vi "mainVI.vi"() -> ()   [LabVIEW 2017]
uses:
  Controls/ShiftRegisterCluster.ctl
  Controls/PhysicalChannelsArray.ctl
  Variables/GlobalData.vi
  <vilib>/regexp/Match Regular Expression.xnode
panel:
  in  "Remote start?":bool
  in  "VRMS simulation?":bool
  in  "VRMS Physical channel":tag caption="Physical channel"
  in  "DI simulation?":bool
  in  "Digital Input Lines":tag
  in  "Temp simulation?":bool
  in  "Temp physical channel":tag caption="Physical channel"
  out "IsAcqGoing":bool
  in  "StopAcqButton":bool
  in  "StartAcqButton":bool
  out "Frequency [Hz]":dbl format="%.2f"
  out "RMS Value [V]":dbl format="%0.2p"
  out "DI data":bool[](array[boolean])
  out "Temperature indicator":dbl caption="Temperature [°C]"
  in  "OK":bool
  # "Temperature"
  # "Digital Inputs"
  # "DAQ"
  # "Sim"
  # "DAQ"
  # "Sim"
  # "Voltage"
  # "DAQ"
  # "Sim"
  # "Remote"
  # "Loclal"
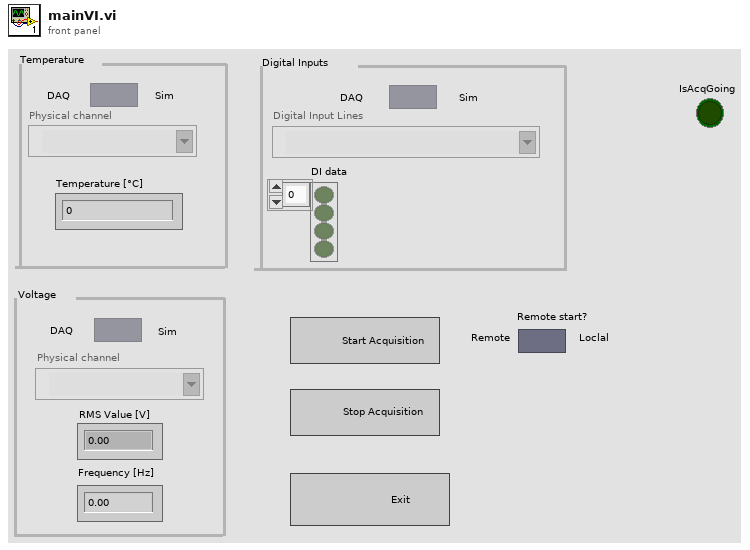
[diagram p1: front panel]
types:
  T1 = enum32{"invalid app kind", "Development System", "Run Time System", "Student Edition", "Embedded LabVIEW", "Evaluation", "Custom"}
  T2 = enum32{"Invalid", "Standard", "Closed", "Hidden", "Minimized", "Maximized"}
  T3 = enum8{"Enabled", "Disabled", "Disabled and Grayed Out"}
  T4 = typedef "ShiftRegisterCluster.ctl" = cluster{"TemperatureTask":refnum<k21>, "TemperatureData":dbl, "EncoderTask":refnum<k21>, "EncoderData":dbl, "DITask":refnum<k21>, "DIData":bool[], "VRMSTask":refnum<k21>, "VRMSData":dbl, "FreqData":dbl}
  T5 = cluster{"TemperatureData":dbl, "DIData":bool[], "VRMSData":dbl, "FreqData":dbl}
  T6 = cluster{"Core":cluster{"Current VI Reference":refnum<vi>, "Close Panel on Exit?":bool}, "Data Cluster":T4, "IsAcqGoing":bool}
  T7 = cluster{"Current VI Reference":refnum<vi>, "Close Panel on Exit?":bool}
  T8 = cluster{"Temp simulation?":bool, "DI simulation?":bool, "VRMS simulation?":bool}
  T9 = cluster{"Temp physical channel":tag, "Digital Input Lines":tag, "VRMS Physical channel":tag}
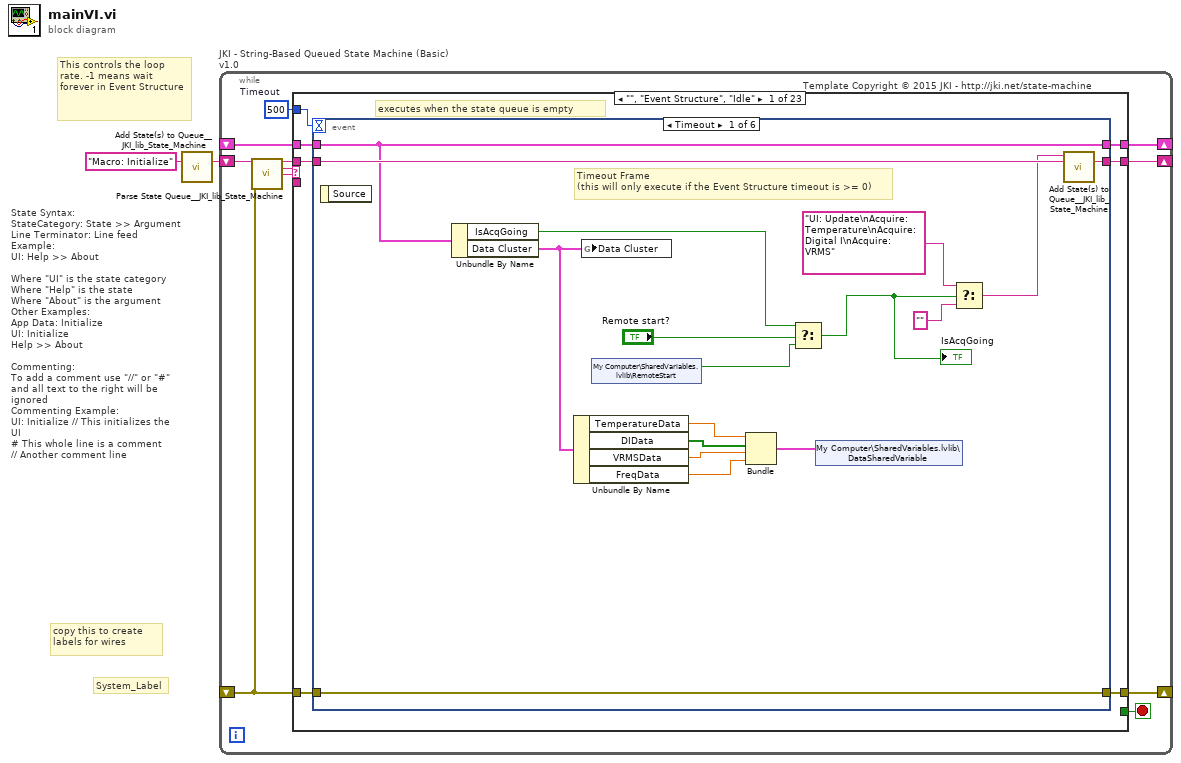
[diagram p0: block diagram]
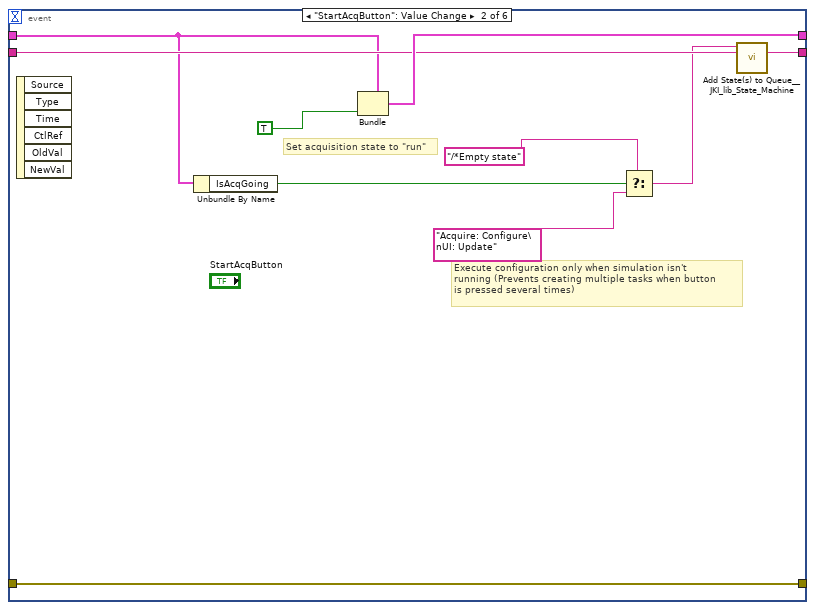
[diagram p2: hidden frame]
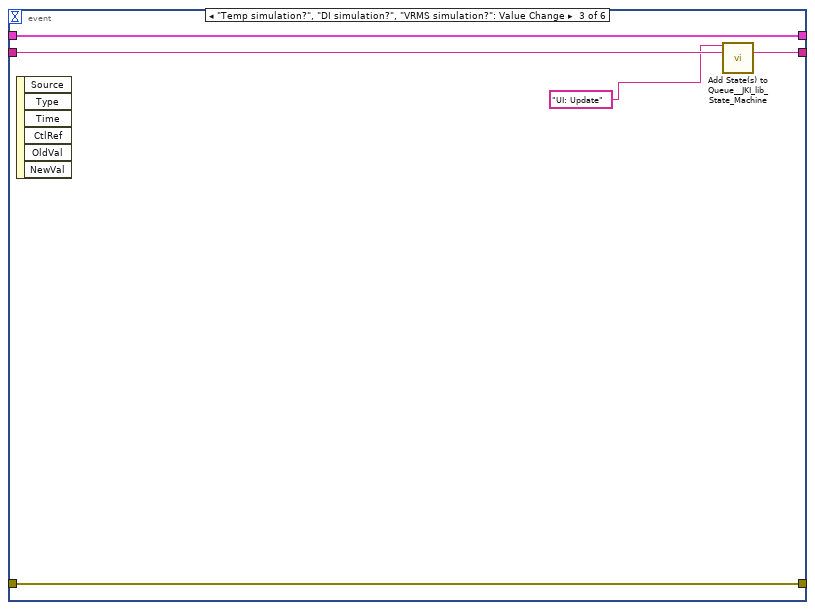
[diagram p3: hidden frame]
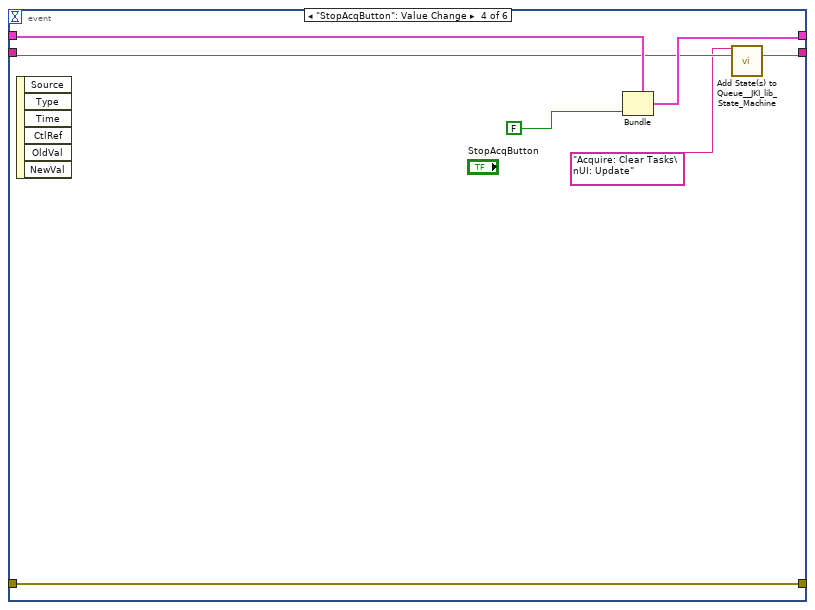
[diagram p4: hidden frame]
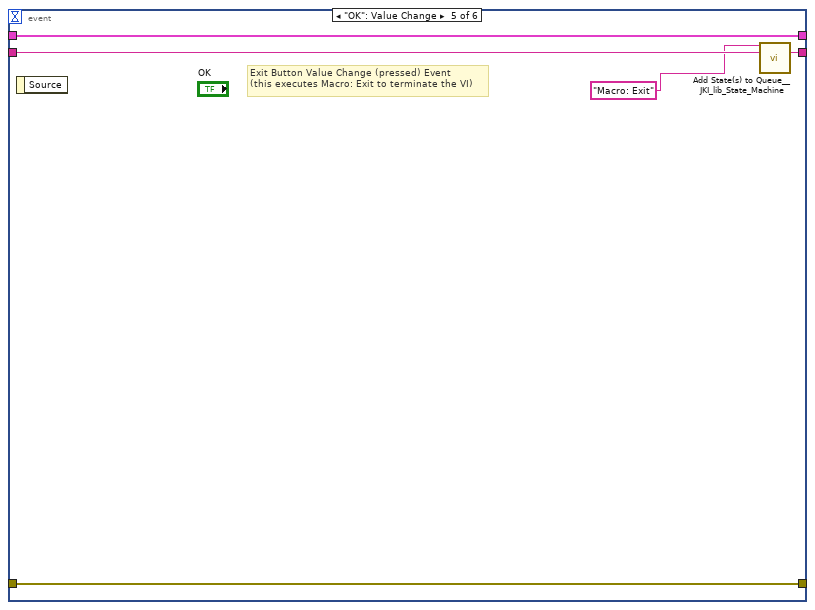
[diagram p5: hidden frame]
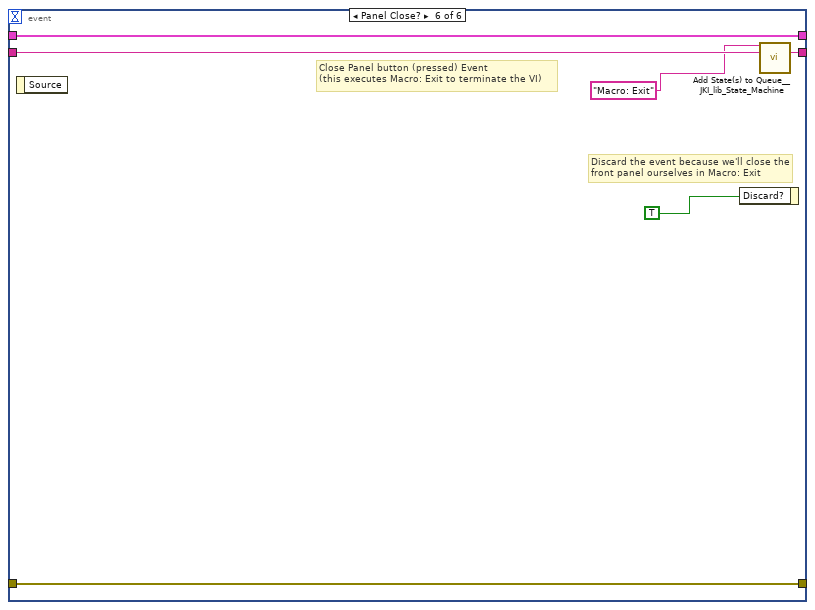
[diagram p6: hidden frame]
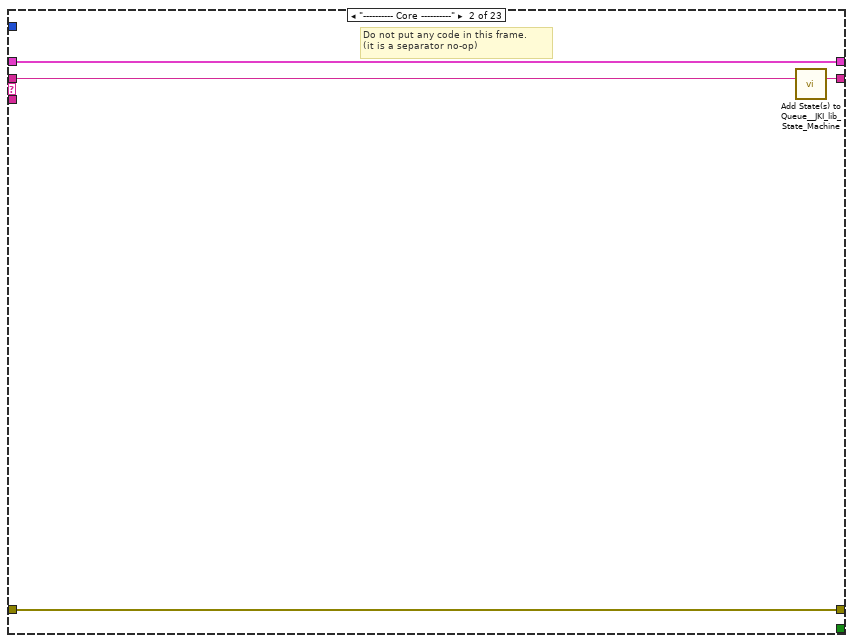
[diagram p7: hidden frame]
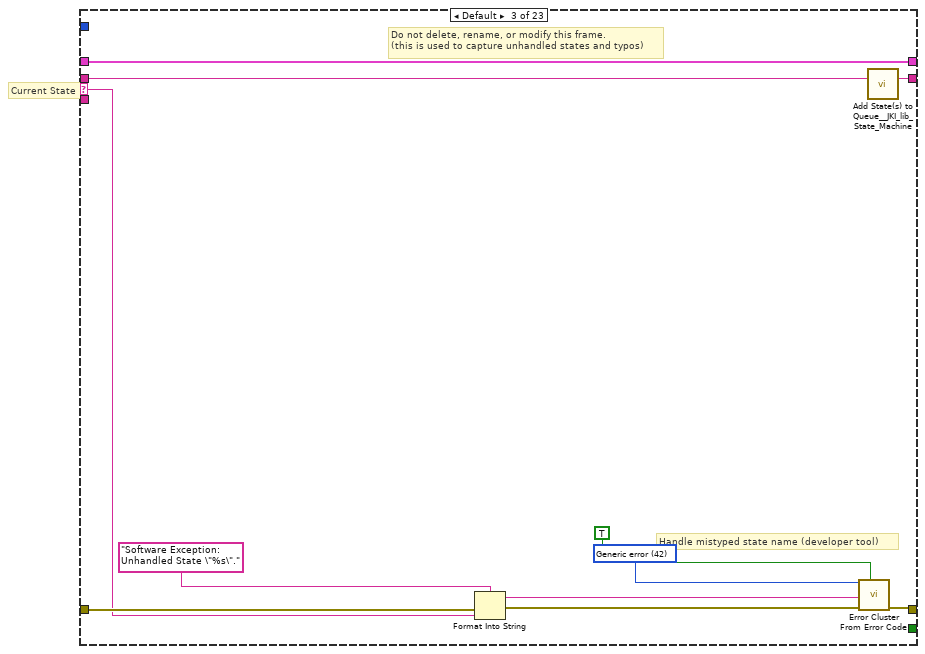
[diagram p8: hidden frame]
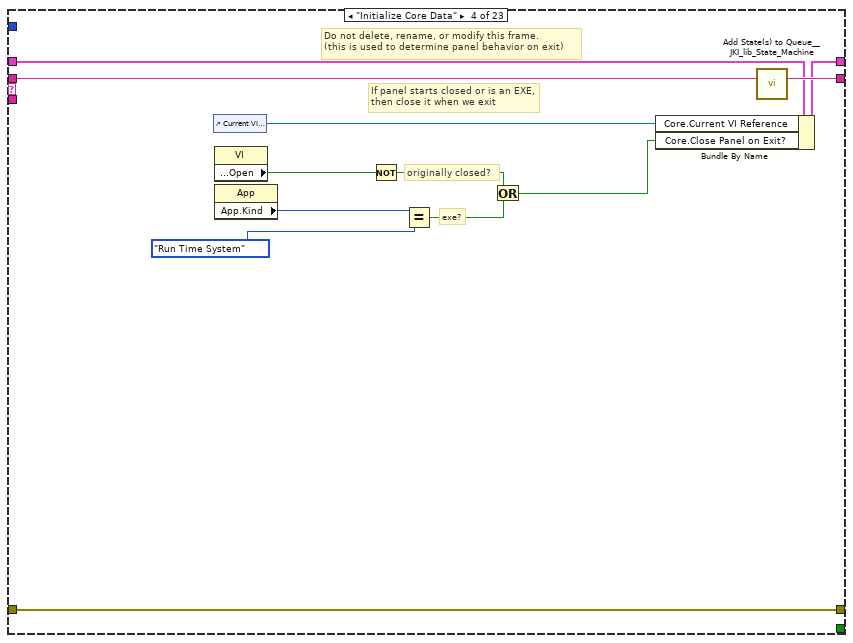
[diagram p9: hidden frame]
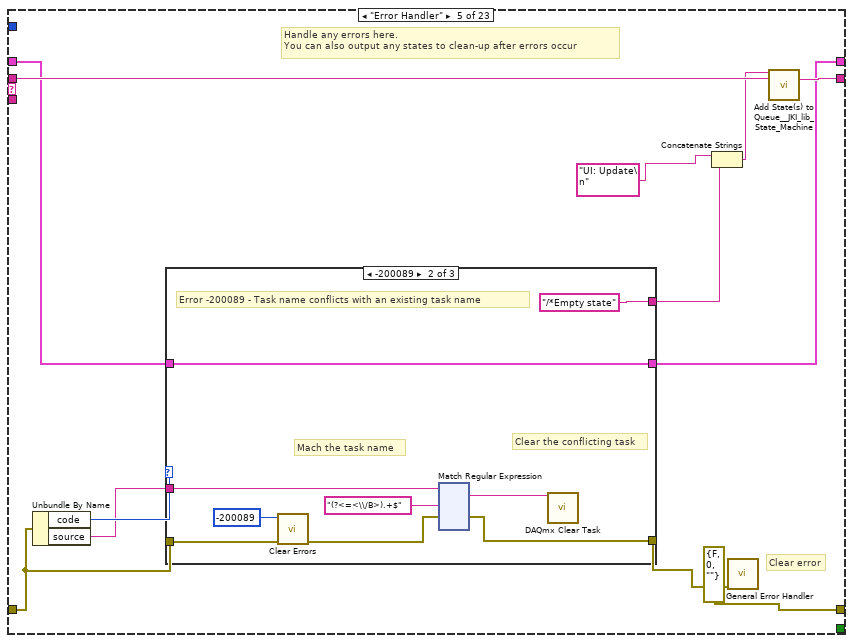
[diagram p10: hidden frame]
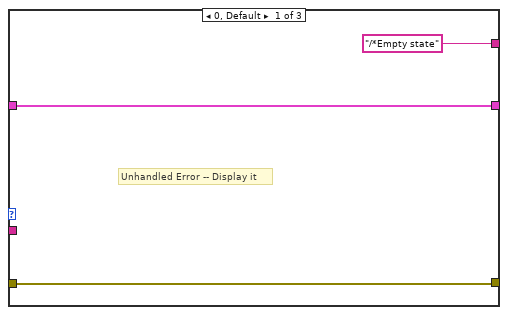
[diagram p11: hidden frame]
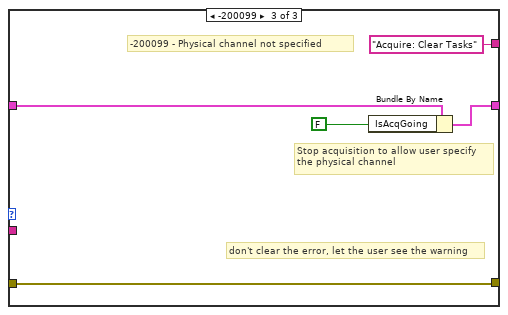
[diagram p12: hidden frame]
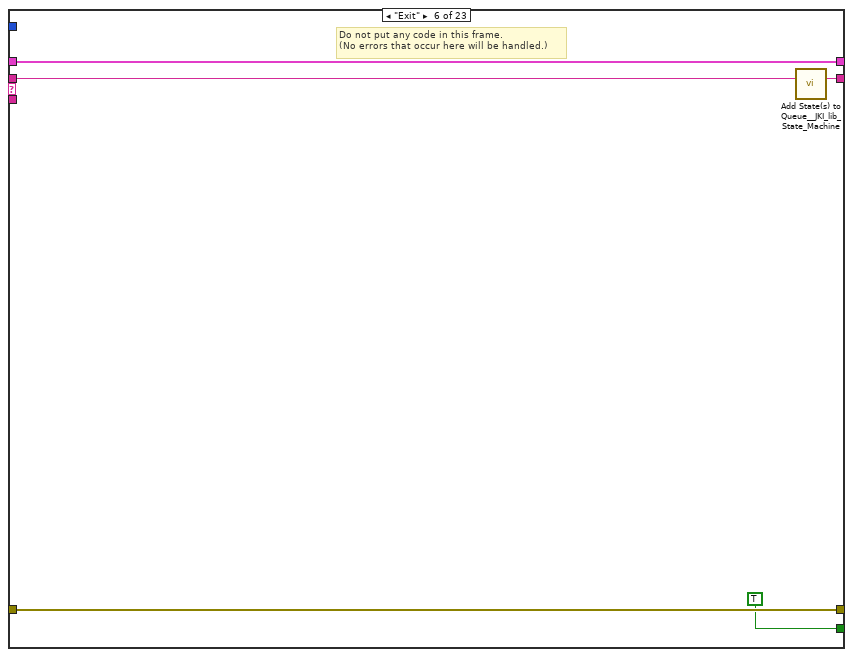
[diagram p13: hidden frame]
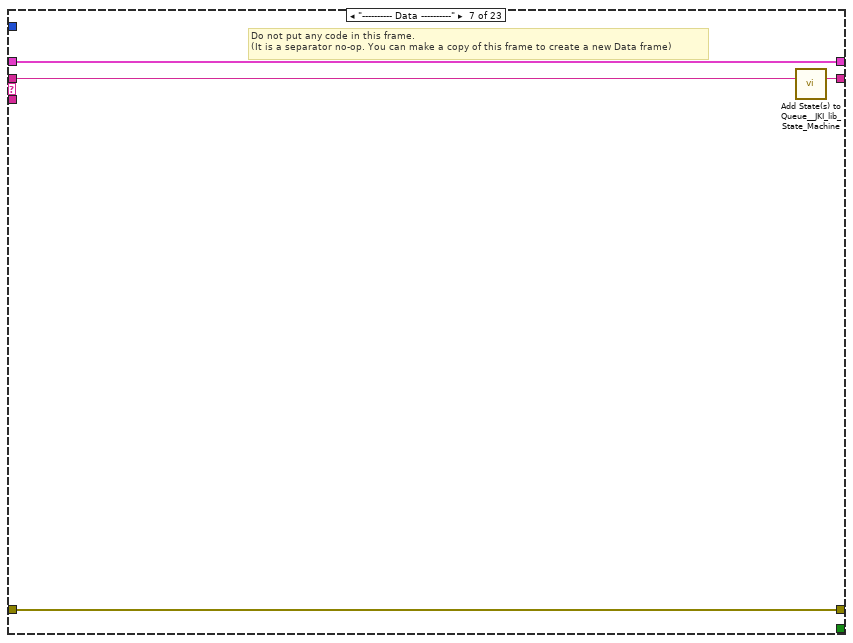
[diagram p14: hidden frame]
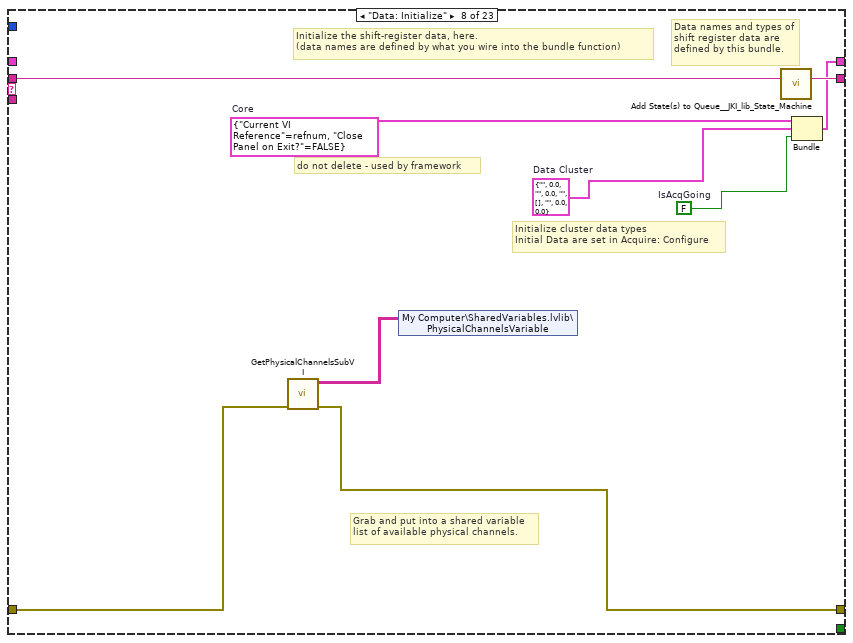
[diagram p15: hidden frame]
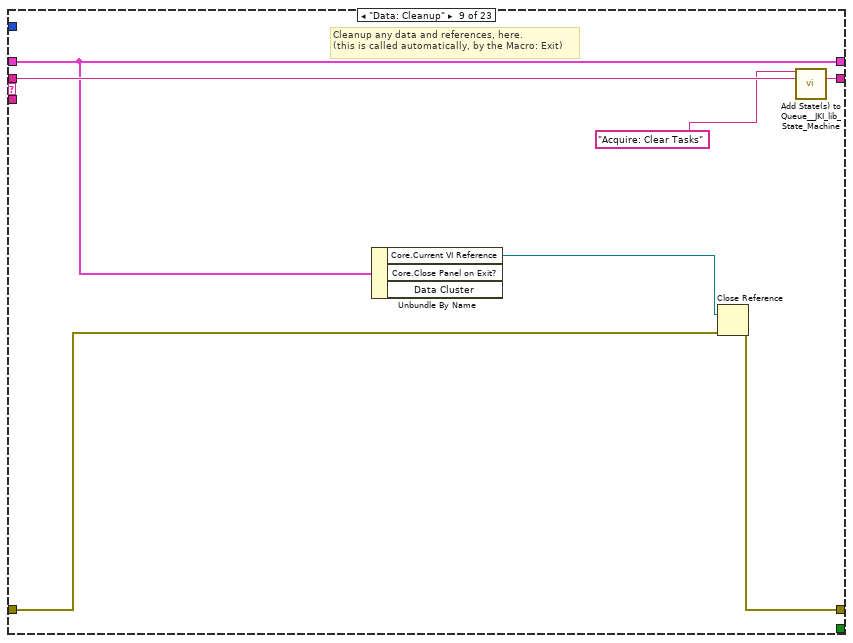
[diagram p16: hidden frame]
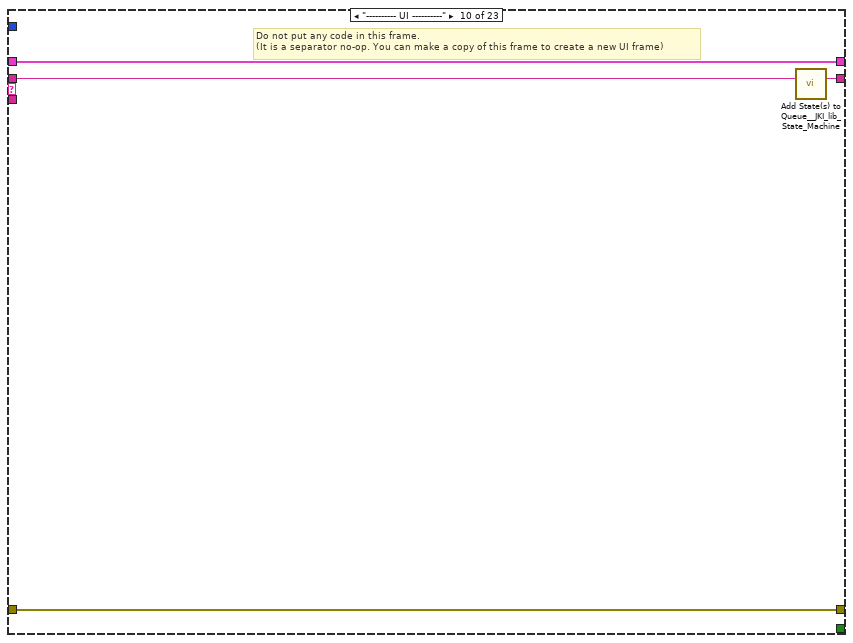
[diagram p17: hidden frame]
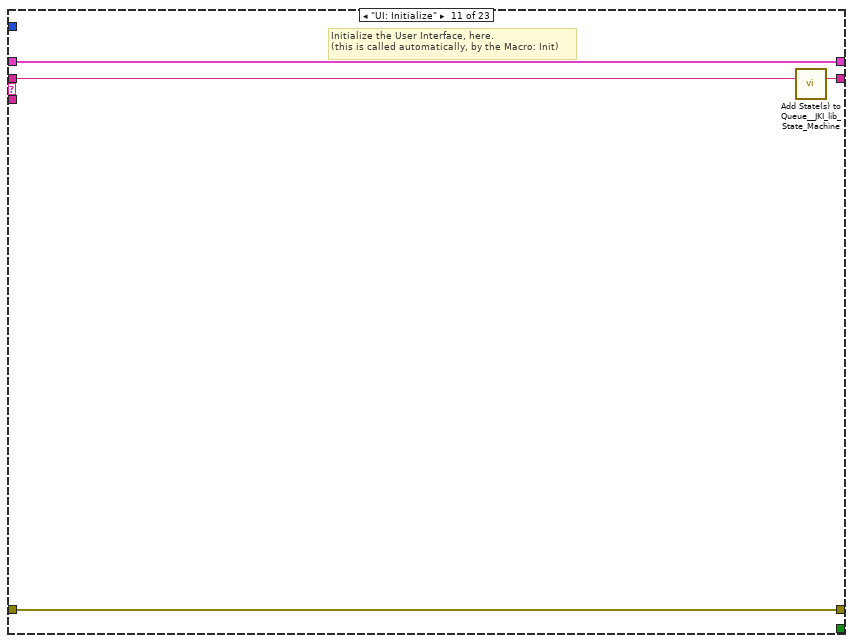
[diagram p18: hidden frame]
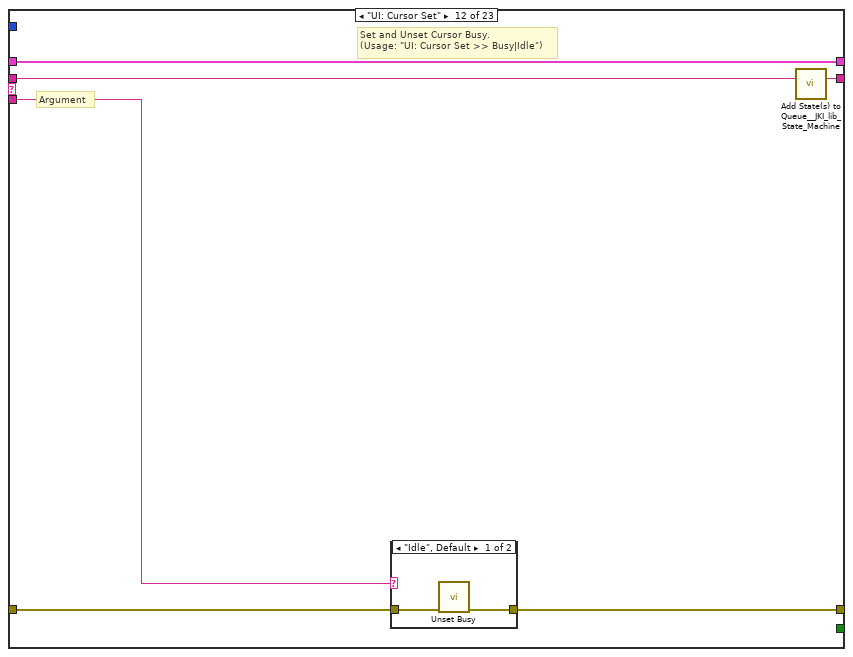
[diagram p19: hidden frame]
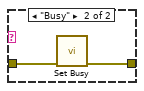
[diagram p20: hidden frame]
diagram:
  # "State Syntax:\nStateCategory: State >> Argument\nLine Terminator: Line feed\nExample:\nUI: Help >> About\n\nWhere \"UI\" is the state category\nWhere \"Help\" is the state\nWhere \"About\" is the argument\nOther Examples:\nApp Data: Initialize\nUI: Initialize\nHelp >> About\n\nCommenting:\nTo add a comment use \"//\" or \"#\" and all text to the right will be ignored\nCommenting Example:\nUI: Initialize // This initializes the UI\n# This whole line is a comment\n// Another comment line"
  # "copy this to create labels for wires"
  # "This controls the loop rate. -1 means wait forever in Event Structure"
  # "System_Label"
  n1 = call <vilib>:"Add State(s) to Queue__JKI_lib_State_Machine.vi"("State(s) in (\"\")"="Macro: Initialize") -> ("States Out"=w2:string)  [unwired: 14 in]
  n2 = while "JKI - String-Based Queued State Machine (Basic) v1.0" {
    shift-right: [w7] -> _
    shift-left: _ -> [w6]
    shift-right: [w3] -> _
    shift-left: _ -> [w4]
    shift-right: [w9] -> _
    shift-left: w2 -> [w10]
    stop <- w8 stop-if-true
    w5 = 500  # Timeout
    # "Template Copyright © 2015 JKI - http://jki.net/state-machine"
    n3 = call <vilib>:"Parse State Queue__JKI_lib_State_Machine.vi"("State Queue"=w10, "Error In (no error)"=w4) -> ("Remaining States"=w12:string, "Current State"=w13:string, "Arguments"=w11:string)  [unwired: 11 in]
    n4 = case shown="\"\", \"Event Structure\", \"Idle\"" w13 {
      selector: w13 -> [_ _ w75 _ _ _ _ _ _ _ _ _ _ _ _ _ _ _ _ _ _ _ _]
      tunnel: w12 -> [w20 w74 w79 w97 w109 w247 w251 w260 w267 w271 w275 w281 w292 w340 w344 w349 w359 w363 w378 w379 w393 w402 w412]
      tunnel: w11 -> [_ _ _ _ _ _ _ _ _ _ _ w276 w286 _ _ _ _ _ _ _ _ _ _]
      tunnel: w6 -> [w18 w71 w77 w88 w102 w245 w248 _ w263 w268 w273 w279 w288 w323 w341 w346 w356 w360 w366 w383 w387 w396 w406]
      tunnel: w4 -> [w16 w72 w80 w94 w104 w244 w249 w254 w262 w269 w272 w278 w290 w318 w342 w347 w357 w361 w368 w380 w391 w400 w410]
      tunnel: [w19 w73 w78 w96 w108 w246 w250 w259 w266 w270 w274 w280 w291 w339 w343 w348 w358 w362 w377 w384 w392 w401 w411] -> w9
      tunnel: [_ _ _ _ _ TRUE _ _ _ _ _ _ _ _ _ _ _ _ _ _ _ _ _] -> w8
      tunnel: [w15 w71 w77 w95 w101 w245 w248 w258 w263 w268 w273 w279 w288 w323 w341 w346 w356 w360 w364 w383 w385 w394 w405] -> w7
      tunnel: w5 -> [w14 _ _ _ _ _ _ _ _ _ _ _ _ _ _ _ _ _ _ _ _ _ _]
      tunnel: [w17 w72 w81 w94 errorcluster {"status"=FALSE, "code"=0, "source"=""} ("error out") w244 w249 w253 w264 w269 w272 w277 w289 w326 w342 w347 w357 w361 w367 w381 w390 w399 w409] -> w3
      frame "", "Event Structure", "Idle" {
        # "executes when the state queue is empty"
        n5 = event shown="[0] Timeout" {
          selector: _ -> [_ _ _ _ _ _]
          dyn-events: _ -> [_ _ _ _ _ _]
          timeout: w14 -> [_ _ _ _ _ _]
          tunnel: w20 -> [w37 w44 w51 w55 w64 w70]
          tunnel: [w36 w45 w52 w56 w63 w69] -> w19
          tunnel: w18 -> [w21 w43 w48 w59 w61 w67]
          tunnel: [w35 w38 w49 w53 w62 w68] -> w17
          tunnel: w16 -> [w35 w38 w49 w53 w62 w68]
          tunnel: [w21 w46 w48 w58 w61 w67] -> w15
          event Timeout {
            # "Timeout Frame\n(this will only execute if the Event Structure timeout is >= 0)"
            n6 = event-data() -> ()  [unwired: 1 in, 1 out]
            n7 = Unbundle By Name(w21) -> ("IsAcqGoing"=w23:bool, "Data Cluster"=w34:T4)
            n8 = Unbundle By Name(w34) -> ("TemperatureData"=w33:dbl, "DIData"=w32:bool[], "VRMSData"=w31:dbl, "FreqData"=w30:dbl)
            n9 = global write "GlobalData.vi" "Data Cluster"(w34) -> ()
            n10 = shared-variable "My Computer\\SharedVariables.lvlib\\RemoteStart"() -> (w24:bool)  [unwired: 1 in, 1 out]
            n11 = Bundle("TemperatureData"=w33, "DIData"=w32, "VRMSData"=w31, "FreqData"=w30) -> (w29:T5)  [unwired: 1 in]
            n12 = Select(t=w23, s="Remote start?", f=w24) -> (s? t:f=w22:bool)
            "IsAcqGoing" <- w22
            n13 = shared-variable "My Computer\\SharedVariables.lvlib\\DataSharedVariable"(w29) -> ()  [unwired: 1 in, 1 out]
            n14 = Select(t="UI: Update\nAcquire: Temperature\nAcquire: Digital I\nAcquire: VRMS" ("State(s) in Front (\"\")"), s=w22, f="") -> (s? t:f=w26:string)
            n15 = call <vilib>:"Add State(s) to Queue__JKI_lib_State_Machine.vi"("State(s) in Front (\"\")"=w26, "State(s) in (\"\")"=w37) -> ("States Out"=w36:string)  [unwired: 13 in]
          }
          event "StartAcqButton": Value Change {
            # "Set acquisition state to \"run\""
            # "Execute configuration only when simulation isn't \nrunning (Prevents creating multiple tasks when button\nis pressed several times)"
            n16 = event-data() -> ()  [unwired: 1 in, 6 out]
            n17 = Unbundle By Name(w43) -> ("IsAcqGoing"=w42:bool)
            n18 = Bundle(cluster=w43, "IsAcqGoing"=TRUE) -> (w46:T6)  [unwired: 2 in]
            n19 = Select(t="/*Empty state", s=w42, f="Acquire: Configure\nUI: Update" ("State(s) in Front (\"\")")) -> (s? t:f=w40:string)
            n20 = call <vilib>:"Add State(s) to Queue__JKI_lib_State_Machine.vi"("State(s) in Front (\"\")"=w40, "State(s) in (\"\")"=w44) -> ("States Out"=w45:string)  [unwired: 13 in]
          }
          event "Temp simulation?", "DI simulation?", "VRMS simulation?": Value Change {
            n21 = event-data() -> ()  [unwired: 1 in, 6 out]
            n22 = call <vilib>:"Add State(s) to Queue__JKI_lib_State_Machine.vi"("State(s) in Front (\"\")"="UI: Update" ("State(s) in Front (\"\")"), "State(s) in (\"\")"=w51) -> ("States Out"=w52:string)  [unwired: 13 in]
          }
          event "StopAcqButton": Value Change {
            n23 = event-data() -> ()  [unwired: 1 in, 6 out]
            n24 = Bundle(cluster=w59, "IsAcqGoing"=FALSE) -> (w58:T6)  [unwired: 2 in]
            n25 = call <vilib>:"Add State(s) to Queue__JKI_lib_State_Machine.vi"("State(s) in Front (\"\")"="Acquire: Clear Tasks\nUI: Update" ("State(s) in Front (\"\")"), "State(s) in (\"\")"=w55) -> ("States Out"=w56:string)  [unwired: 13 in]
          }
          event "OK": Value Change {
            # "Exit Button Value Change (pressed) Event\n(this executes Macro: Exit to terminate the VI)"
            n26 = event-data() -> ()  [unwired: 1 in, 1 out]
            n27 = call <vilib>:"Add State(s) to Queue__JKI_lib_State_Machine.vi"("State(s) in Front (\"\")"="Macro: Exit", "State(s) in (\"\")"=w64) -> ("States Out"=w63:string)  [unwired: 13 in]
          }
          event Panel Close? {
            # "Discard the event because we'll close the front panel ourselves in Macro: Exit"
            # "Close Panel button (pressed) Event\n(this executes Macro: Exit to terminate the VI)"
            n28 = event-data() -> ()  [unwired: 1 in, 1 out]
            n29 = event-data("Discard?"=TRUE) -> ()  [unwired: 1 in, 1 out]
            n30 = call <vilib>:"Add State(s) to Queue__JKI_lib_State_Machine.vi"("State(s) in Front (\"\")"="Macro: Exit", "State(s) in (\"\")"=w70) -> ("States Out"=w69:string)  [unwired: 13 in]
          }
        }
      }
      frame "---------- Core ----------" {
        # "Do not put any code in this frame.\n(it is a separator no-op)"
        n31 = call <vilib>:"Add State(s) to Queue__JKI_lib_State_Machine.vi"("State(s) in (\"\")"=w74) -> ("States Out"=w73:string)  [unwired: 14 in]
      }
      frame Default {
        w84 = 42 items=["No error", "Argument error", "Memory is full", "Out of zone", "End of file", "File already open", "Generic file I/O error", "File not found", "File permission error", "Disk is full", "Duplicate path", "Too many files open", "System feature not enabled", "Resource file not found", "Cannot add resource", "Resource not found", "Image not found", "Image memory error", "Pen does not exist", "Config type invalid", "Config token not found", "Config parse error", "Config memory error", "Bad external code format", "Bad external code offset", "External code not present", "Null window", "Destroy window error", "Null menu", "Print aborted", "Bad print record", "Print driver error", "Windows error during printing", "Memory error during printing", "Print dialog error", "Generic print error", "Invalid device refnum", "Device not found", "Device parameter error", "Device unit error", "Cannot open device", "Device call aborted", "Generic error", "Cancelled by user", "Object ID too low", "Object ID too high", "Object not in heap", "Unknown heap", "Unknown object (invalid DefProc)", "Unknown object (DefProc not in table)", "Message out of range", "Invalid (null) method", "Unknown message", "Manager call not supported", "Bad address", "Network operation in progress", "Network operation timed out", "Connection is busy", "Network attribute not supported", "Network error", "Address in use", "System out of memory", "Connection aborted", "Connection refused", "Not connected", "Already connected", "Connection closed", "Initialization error (interapplication manager)", "Bad occurrence", "Wait on unbound occurrence handler", "Occurrence queue overflow", "Datalog type conflict", "Unused", "Unrecognized type (interapplication manager)", "Memory corrupt", "Failed to make temporary DLL", "Old CIN version", "Drag socket not found", "Failed to load drop-object", "Failed to register OLE object", "Failed to release OLE object", "Format specifier type mismatch", "Unknown format specifier", "Too few format specifiers", "Too many format specifiers", "Scan failed", "Newer CIN version", "Error converting to variant", "Runtime menu error", "Password tampered", "Variant attribute not found", "Incompatible variant data type", "Event data is not available", "Event Store is not present", "Occurrence is not found", "Event Queue is not created", "Event info is not available", "Refnum passed is NULL", "Error retrieving Class GUID", "Error retrieving CoClass GUID", "Error retrieving TypeLib GUID.", "Bad built application magic bytes.", "Specific driver is different from the specific driver associated with the Logical Name.", "There is no session opened to the class driver.", "Max Error", "MAX - Error with config objects", "MAX - Error loading configuration", "MAX - Group not supported"]
        # "Current State"
        # "Do not delete, rename, or modify this frame.\n(this is used to capture unhandled states and typos)"
        # "Handle mistyped state name (developer tool)"
        n32 = Format Into String(format string="Software Exception: Unhandled State \"%s\"." ("message"), error in=w80, w75) -> (resulting string=w83:string, error out=w82:errorcluster)  [unwired: 1 in]
        n33 = call <vilib>:"Error Cluster From Error Code.vi"("show call chain? (False)"=TRUE, "error in (no error)"=w82, "error message (\"\")"=w83, "error code (0)"=w84) -> ("error out"=w81:errorcluster)  [unwired: 5 in]
        n34 = call <vilib>:"Add State(s) to Queue__JKI_lib_State_Machine.vi"("State(s) in (\"\")"=w79) -> ("States Out"=w78:string)  [unwired: 14 in]
      }
      frame "Initialize Core Data" {
        # "Do not delete, rename, or modify this frame.\n(this is used to determine panel behavior on exit)"
        # "originally closed?"
        # "exe?"
        # "If panel starts closed or is an EXE, then close it when we exit"
        n35 = control-ref of="Current VI Reference"() -> (w86:refnum<vi>)
        n36 = property class="VI"() -> ("Front Panel.Open"=w93:bool)  [unwired: 2 in, 2 out]
        n37 = property class="App"() -> ("App.Kind"=w92:T1)  [unwired: 2 in, 2 out]
        n38 = Not(x=w93) -> (.not. x?=w90:bool)
        n39 = Equal?(x=w92, y=T1."Run Time System" ("Application:Kind")) -> (x = y?=w89:bool)
        n40 = Or(x=w90, y=w89) -> (x .or. y?=w87:bool)
        n41 = Bundle By Name(cluster=w88, "Core.Current VI Reference"=w86, "Core.Close Panel on Exit?"=w87) -> (w95:T6)
        n42 = call <vilib>:"Add State(s) to Queue__JKI_lib_State_Machine.vi"("State(s) in (\"\")"=w97) -> ("States Out"=w96:string)  [unwired: 14 in]
      }
      frame "Error Handler" {
        # "Handle any errors here.\nYou can also output any states to clean-up after errors occur"
        # "Clear error"
        n43 = Unbundle By Name(w104) -> ("code"=w106:i32, "source"=w105:string)
        n44 = case shown="-200089" w106 {
          tunnel: w105 -> [_ w121 _]
          tunnel: w104 -> [w112 w118 w238]
          tunnel: [w112 w115 w238] -> w103
          tunnel: w102 -> [w111 w114 w242]
          tunnel: [w111 w114 w240] -> w101
          tunnel: ["/*Empty state" "/*Empty state" "Acquire: Clear Tasks"] -> w100
          frame 0, Default {
            # "Unhandled Error -- Display it"
          }
          frame -200089 {
            # "Mach the task name"
            # "Clear the conflicting task"
            # "Error -200089 - Task name conflicts with an existing task name"
            n45 = call <vilib>:"Clear Errors.vi"("error in (no error)"=w118, "specific error code to clear (0: all)"=-200089) -> ("error out"=w117:errorcluster)  [unwired: 4 in, 1 out]
            n46 = xnode "Match Regular Expression"("input string"=w121, "regular expression"="(?<=<\\/B>).+$", "error in"=w117) -> ("whole match"=w119:string, "error out"=w115:errorcluster)  [unwired: 3 in, 4 out]
            n47 = call <vilib>:"DAQmx Clear Task.vi"("task in"=w119) -> ()  [unwired: 14 in, 1 out]
          }
          frame -200099 {
            # "don't clear the error, let the user see the warning"
            # "Stop acquisition to allow user specify\nthe physical channel"
            # "-200099 - Physical channel not specified"
            n48 = Bundle By Name(cluster=w242, "IsAcqGoing"=FALSE) -> (w240:T6)
          }
        }
        n49 = Concatenate Strings("UI: Update\n" ("string"), w100) -> (w98:string)
        n50 = call <vilib>:"General Error Handler.vi"("error in (no error)"=w103) -> ()  [unwired: 10 in, 5 out]
        n51 = call <vilib>:"Add State(s) to Queue__JKI_lib_State_Machine.vi"("State(s) in Front (\"\")"=w98, "State(s) in (\"\")"=w109) -> ("States Out"=w108:string)  [unwired: 13 in]
      }
      frame "Exit" {
        # "Do not put any code in this frame.\n(No errors that occur here will be handled.)"
        n52 = call <vilib>:"Add State(s) to Queue__JKI_lib_State_Machine.vi"("State(s) in (\"\")"=w247) -> ("States Out"=w246:string)  [unwired: 14 in]
      }
      frame "---------- Data ----------" {
        # "Do not put any code in this frame.\n(It is a separator no-op. You can make a copy of this frame to create a new Data frame)"
        n53 = call <vilib>:"Add State(s) to Queue__JKI_lib_State_Machine.vi"("State(s) in (\"\")"=w251) -> ("States Out"=w250:string)  [unwired: 14 in]
      }
      frame "Data: Initialize" {
        w255 = FALSE  # IsAcqGoing
        w256 = T4 {"TemperatureTask"="", "TemperatureData"=0.0, "EncoderTask"="", "EncoderData"=0.0, "DITask"="", "DIData"=[], "VRMSTask"="", "VRMSData"=0.0, "FreqData"=0.0}  # Data Cluster
        w257 = T7 {"Current VI Reference"=refnum, "Close Panel on Exit?"=FALSE}  # Core
        # "Grab and put into a shared variable\nlist of available physical channels."
        # "Initialize cluster data types\nInitial Data are set in Acquire: Configure"
        # "do not delete - used by framework"
        # "Data names and types of shift register data are defined by this bundle."
        # "Initialize the shift-register data, here.\n(data names are defined by what you wire into the bundle function)"
        n54 = call "GetPhysicalChannelsSubVI.vi"("error in (no error)"=w254) -> ("error out"=w253:errorcluster, "Physical Channels"=w252:string[][])  [unwired: 9 in]
        n55 = shared-variable "My Computer\\SharedVariables.lvlib\\PhysicalChannelsVariable"(w252) -> ()  [unwired: 1 in, 1 out]
        n56 = call <vilib>:"Add State(s) to Queue__JKI_lib_State_Machine.vi"("State(s) in (\"\")"=w260) -> ("States Out"=w259:string)  [unwired: 14 in]
        n57 = Bundle("Core"=w257, "Data Cluster"=w256, "IsAcqGoing"=w255) -> (w258:T6)  [unwired: 1 in]
      }
      frame "Data: Cleanup" {
        # "Cleanup any data and references, here.\n(this is called automatically, by the Macro: Exit)"
        n58 = Unbundle By Name(w263) -> ("Core.Current VI Reference"=w265:refnum<vi>)  [unwired: 2 out]
        n59 = Close Reference(reference=w265, error in (no error)=w262) -> (error out=w264:errorcluster)
        n60 = call <vilib>:"Add State(s) to Queue__JKI_lib_State_Machine.vi"("State(s) in Front (\"\")"="Acquire: Clear Tasks" ("State(s) in Front (\"\")"), "State(s) in (\"\")"=w267) -> ("States Out"=w266:string)  [unwired: 13 in]
      }
      frame "---------- UI ----------" {
        # "Do not put any code in this frame.\n(It is a separator no-op. You can make a copy of this frame to create a new UI frame)"
        n61 = call <vilib>:"Add State(s) to Queue__JKI_lib_State_Machine.vi"("State(s) in (\"\")"=w271) -> ("States Out"=w270:string)  [unwired: 14 in]
      }
      frame "UI: Initialize" {
        # "Initialize the User Interface, here.\n(this is called automatically, by the Macro: Init)"
        n62 = call <vilib>:"Add State(s) to Queue__JKI_lib_State_Machine.vi"("State(s) in (\"\")"=w275) -> ("States Out"=w274:string)  [unwired: 14 in]
      }
      frame "UI: Cursor Set" {
        # "Argument"
        # "Set and Unset Cursor Busy.\n(Usage: \"UI: Cursor Set >> Busy|Idle\")"
        n63 = case shown="\"Idle\", Default" w276 {
          tunnel: w278 -> [w283 w285]
          tunnel: [w282 w284] -> w277
          frame "Idle", Default {
            n64 = call <vilib>:"Unset Busy.vi"("error in (no error)"=w283) -> ("error out"=w282:errorcluster)  [unwired: 10 in]
          }
          frame "Busy" {
            n65 = call <vilib>:"Set Busy.vi"("error in (no error)"=w285) -> ("error out"=w284:errorcluster)  [unwired: 9 in, 1 out]
          }
        }
        n66 = call <vilib>:"Add State(s) to Queue__JKI_lib_State_Machine.vi"("State(s) in (\"\")"=w281) -> ("States Out"=w280:string)  [unwired: 14 in]
      }
      frame "UI: Front Panel State" {
        # "Argument"
        # "Set Front Panel Open or Closed\n(Usage: \"UI: Front Panel State >> Open|Close\")"
        n67 = Unbundle By Name(w288) -> ("Core.Current VI Reference"=w287:refnum<vi>)
        n68 = case shown="\"Open\", Default" w286 {
          tunnel: w290 -> [w296 w309]
          tunnel: [w298 w310] -> w289
          tunnel: w287 -> [w297 w307]
          frame "Open", Default {
            n69 = property class="VI"(reference=w297, error in=w296) -> (reference out=w294:refnum<vi>, error out=w295:errorcluster, "Front Panel.Open"=w293:bool)
            n70 = case shown="True" w293 {
              tunnel: [w301 w304] -> w298
              tunnel: w295 -> [w300 w304]
              tunnel: w294 -> [w299 _]
              frame False {
                n71 = invoke class="VI" method="FP.Open"(reference=w299, error in=w300, "Activate"=TRUE, "State"=T2."Standard") -> (error out=w301:errorcluster)  [unwired: 1 in, 4 out]
              }
              frame True {
              }
            }
          }
          frame "Close" {
            n72 = property class="VI"(reference=w307, error in=w309) -> (reference out=w306:refnum<vi>, error out=w308:errorcluster, "Front Panel.Open"=w305:bool)
            n73 = case shown="True" w305 {
              tunnel: [w311 w314] -> w310
              tunnel: w308 -> [w311 w313]
              tunnel: w306 -> [_ w312]
              frame False {
              }
              frame True {
                n74 = invoke class="VI" method="FP.Close"(reference=w312, error in=w313) -> (error out=w314:errorcluster)  [unwired: 1 in, 2 out]
              }
            }
          }
        }
        n75 = call <vilib>:"Add State(s) to Queue__JKI_lib_State_Machine.vi"("State(s) in (\"\")"=w292) -> ("States Out"=w291:string)  [unwired: 14 in]
      }
      frame "UI: Update" {
        w324 = T3."Enabled" ("Disabled")
        w325 = T3."Disabled and Grayed Out" ("Disabled")
        # "Disable sim/DAQ switch when simulation is running"
        # "Disable channel selection if simulation option is selected"
        n76 = Unbundle By Name(w323) -> ("IsAcqGoing"=w322:bool)
        n77 = property on="VRMS simulation?" class="Bool (strict)"(error in=w318) -> (error out=w330:errorcluster, "Value"=w336:bool)  [unwired: 1 in, 1 out]
        n78 = property on="DI simulation?" class="Bool (strict)"(error in=w318) -> (error out=w331:errorcluster, "Value"=w337:bool)  [unwired: 1 in, 1 out]
        n79 = property on="Temp simulation?" class="Bool (strict)"(error in=w318) -> (error out=w332:errorcluster, "Value"=w338:bool)  [unwired: 1 in, 1 out]
        n80 = Select(t=T3."Disabled and Grayed Out" ("Disabled"), s=w322, f=T3."Enabled" ("Disabled")) -> (s? t:f=w319:T3)
        n81 = Select(t=w325, s=w338, f=w324) -> (s? t:f=w333:T3)
        n82 = Select(t=w325, s=w337, f=w324) -> (s? t:f=w334:T3)
        n83 = Select(t=w325, s=w336, f=w324) -> (s? t:f=w335:T3)
        n84 = property on="VRMS simulation?" class="Bool (strict)"(error in=w318, "DisabledEnum"=w319) -> (error out=w315:errorcluster)  [unwired: 1 in, 1 out]
        n85 = property on="DI simulation?" class="Bool (strict)"(error in=w318, "DisabledEnum"=w319) -> (error out=w316:errorcluster)  [unwired: 1 in, 1 out]
        n86 = property on="Temp simulation?" class="Bool (strict)"(error in=w318, "DisabledEnum"=w319) -> (error out=w317:errorcluster)  [unwired: 1 in, 1 out]
        n87 = property on="Temp physical channel" class="DAQmxName"(error in=w332, "DisabledEnum"=w333) -> (error out=w329:errorcluster)  [unwired: 1 in, 1 out]
        n88 = property on="VRMS Physical channel" class="DAQmxName"(error in=w330, "DisabledEnum"=w335) -> (error out=w327:errorcluster)  [unwired: 1 in, 1 out]
        n89 = property on="Digital Input Lines" class="DAQmxName"(error in=w331, "DisabledEnum"=w334) -> (error out=w328:errorcluster)  [unwired: 1 in, 1 out]
        n90 = Merge Errors(w317, w316, w315, w329, w328, w327) -> (w326:errorcluster)
        n91 = call <vilib>:"Add State(s) to Queue__JKI_lib_State_Machine.vi"("State(s) in (\"\")"=w340) -> ("States Out"=w339:string)  [unwired: 14 in]
      }
      frame "---------- Macro ----------" {
        # "Do not put any code in this frame.\n(It is a separator no-op. You can make a copy of this frame to create a new Macro frame)"
        n92 = call <vilib>:"Add State(s) to Queue__JKI_lib_State_Machine.vi"("State(s) in (\"\")"=w344) -> ("States Out"=w343:string)  [unwired: 14 in]
      }
      frame "Macro: Initialize" {
        w345 = "Data: Initialize\nInitialize Core Data\nUI: Initialize\nUI: Front Panel State >> Open\nUI: Update"  # Data: Initialize Initialize Core Data UI: Initialize UI: Front Panel State >> Open UI: Update
        # "Initialization Macro\n(This is called once, when the VI starts)"
        n93 = call <vilib>:"Add State(s) to Queue__JKI_lib_State_Machine.vi"("State(s) in Front (\"\")"=w345, "State(s) in (\"\")"=w349) -> ("States Out"=w348:string)  [unwired: 13 in]
      }
      frame "Macro: Exit" {
        # "Exit Macro\n(This is called once, when the VI exits)"
        n94 = Unbundle By Name(w356) -> ("Core.Close Panel on Exit?"=w355:bool)
        n95 = Select(t="UI: Front Panel State >> Close", s=w355, f="") -> (s? t:f=w352:string)
        n96 = call <vilib>:"Add State(s) to Queue__JKI_lib_State_Machine.vi"("State(s) in (\"\")"=w352, "State(s) at Back (\"\")"="Data: Cleanup\nExit") -> ("States Out"=w350:string)  [unwired: 13 in]
        n97 = call <vilib>:"Add State(s) to Queue__JKI_lib_State_Machine.vi"("State(s) in Front (\"\")"=w350, "State(s) in (\"\")"=w359) -> ("States Out"=w358:string)  [unwired: 13 in]
      }
      frame "---------- Acquire ----------" {
        # "Template Separator\n(You can make a copy of, or modify, this frame)"
        n98 = call <vilib>:"Add State(s) to Queue__JKI_lib_State_Machine.vi"("State(s) in (\"\")"=w363) -> ("States Out"=w362:string)  [unwired: 14 in]
      }
      frame "Acquire: Configure" {
        n99 = Bundle("Temp simulation?"="Temp simulation?", "DI simulation?"="DI simulation?", "VRMS simulation?"="VRMS simulation?") -> (w369:T8)  [unwired: 1 in]
        n100 = Bundle("Temp physical channel"="Temp physical channel", "Digital Input Lines"="Digital Input Lines", "VRMS Physical channel"="VRMS Physical channel") -> (w370:T9)  [unwired: 1 in]
        n101 = call "ConfigurationSubVI.vi"("error in (no error)"=w368, "Sim? Cluster"=w369, "Channels Cluster"=w370) -> ("error out"=w367:errorcluster, "Data Cluster"=w365:T4)  [unwired: 7 in]
        n102 = Bundle By Name(cluster=w366, "Data Cluster"=w365) -> (w364:T6)
        n103 = call <vilib>:"Add State(s) to Queue__JKI_lib_State_Machine.vi"("State(s) in (\"\")"=w378) -> ("States Out"=w377:string)  [unwired: 14 in]
      }
      frame "Acquire: Clear Tasks" {
        # "Template Separator\n(You can make a copy of, or modify, this frame)"
        n104 = Unbundle By Name(w383) -> ("Data Cluster"=w382:T4)
        n105 = call "Clear_DAQ_Tasks.vi"("error in (no error)"=w380, "Data Cluster"=w382) -> ("error out"=w381:errorcluster)  [unwired: 9 in]
        n106 = call <vilib>:"Add State(s) to Queue__JKI_lib_State_Machine.vi"("State(s) in (\"\")"=w379) -> ("States Out"=w384:string)  [unwired: 14 in]
      }
      frame "Acquire: Temperature" {
        n107 = Unbundle By Name(w387) -> ("Data Cluster"=w388:T4)
        n108 = call "TempAcqSubVI.vi"("error in (no error)"=w391, "Data Cluster in"=w388) -> ("error out"=w390:errorcluster, "Temperature"=→"Temperature indicator":dbl, "Data Cluster out"=w386:T4)  [unwired: 7 in]
        n109 = Bundle By Name(cluster=w387, "Data Cluster"=w386) -> (w385:T6)
        n110 = call <vilib>:"Add State(s) to Queue__JKI_lib_State_Machine.vi"("State(s) in (\"\")"=w393) -> ("States Out"=w392:string)  [unwired: 14 in]
      }
      frame "Acquire: Digital I" {
        n111 = Unbundle By Name(w396) -> ("Data Cluster"=w397:T4)
        n112 = call "DIAcqSubVI.vi"("error in (no error)"=w400, "Data Cluster In"=w397) -> ("error out"=w399:errorcluster, "data"=→"DI data":bool[], "Data Cluster Out"=w395:T4)  [unwired: 7 in]
        n113 = Bundle By Name(cluster=w396, "Data Cluster"=w395) -> (w394:T6)
        n114 = call <vilib>:"Add State(s) to Queue__JKI_lib_State_Machine.vi"("State(s) in (\"\")"=w402) -> ("States Out"=w401:string)  [unwired: 14 in]
      }
      frame "Acquire: VRMS" {
        n115 = Unbundle By Name(w406) -> ("Data Cluster"=w408:T4)
        n116 = call "VRMSFreqAcqSubVI.vi"("error in (no error)"=w410, "Data Cluster in"=w408) -> ("error out"=w409:errorcluster, "freq"=→"Frequency [Hz]":dbl, "RMS value"=→"RMS Value [V]":dbl, "Data Cluster out"=w407:T4)  [unwired: 6 in]
        n117 = Bundle By Name(cluster=w406, "Data Cluster"=w407) -> (w405:T6)
        n118 = call <vilib>:"Add State(s) to Queue__JKI_lib_State_Machine.vi"("State(s) in (\"\")"=w412) -> ("States Out"=w411:string)  [unwired: 14 in]
      }
    }
  }
